vi "状态标记位读写.vi"(5 "更新状态？":bool, 7 "Slave ID":T2=enum."氨氮", 11 "状态":bool) -> (3 "流程运行状态标记位":T1)   [LabVIEW 2016, in "质控单元V4.lvlib"]
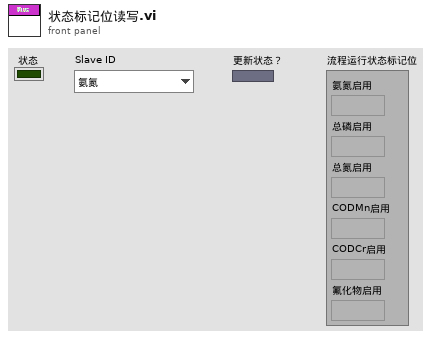
[diagram p1: front panel]
types:
  T1 = typedef "质控单元V4.lvlib/启动参数.ctl" = cluster{"氨氮启用":bool, "总磷启用":bool, "总氮启用":bool, "CODMn启用":bool, "CODCr启用":bool, "氟化物启用":bool}
  T2 = typedef "质控单元V4.lvlib/质控slave id.ctl" = enum16{"null", "氨氮", "总磷", "总氮", "CODMn", "CODCr", "氟化物", "挥发酚"}
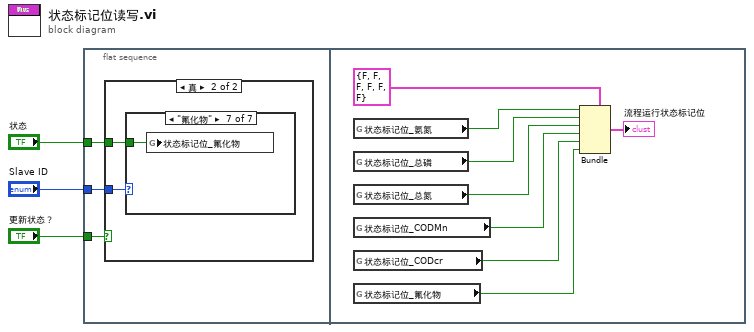
[diagram p0: block diagram]
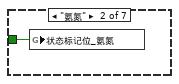
[diagram p4: hidden frame]
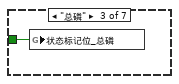
[diagram p5: hidden frame]
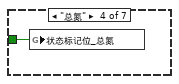
[diagram p6: hidden frame]
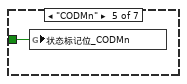
[diagram p7: hidden frame]
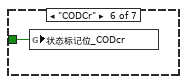
[diagram p8: hidden frame]
diagram:
  n1 = flat-sequence {
    tunnel: "Slave ID" -> [w6]
    tunnel: "状态" -> [w5]
    tunnel: "更新状态？" -> [w4]
    frame #0 {
      n2 = case shown="真" w4 {
        tunnel: w6 -> [_ w8]
        tunnel: w5 -> [_ w7]
        frame False {
        }
        frame True {
          n3 = case shown="\"氟化物\"" w8 {
            tunnel: w7 -> [_ w9 w10 w11 w12 w13 w14]
            frame "null", Default {
            }
            frame "氨氮" {
              n4 = global write "ZK非断电保存全局变量.vi" "状态标记位_氨氮"(w9) -> ()
            }
            frame "总磷" {
              n5 = global write "ZK非断电保存全局变量.vi" "状态标记位_总磷"(w10) -> ()
            }
            frame "总氮" {
              n6 = global write "ZK非断电保存全局变量.vi" "状态标记位_总氮"(w11) -> ()
            }
            frame "CODMn" {
              n7 = global write "ZK非断电保存全局变量.vi" "状态标记位_CODMn"(w12) -> ()
            }
            frame "CODCr" {
              n8 = global write "ZK非断电保存全局变量.vi" "状态标记位_CODcr"(w13) -> ()
            }
            frame "氟化物" {
              n9 = global write "ZK非断电保存全局变量.vi" "状态标记位_氟化物"(w14) -> ()
            }
          }
        }
      }
    }
    frame #1 {
      n10 = global read "ZK非断电保存全局变量.vi" "状态标记位_氨氮"() -> (w22:bool)
      n11 = global read "ZK非断电保存全局变量.vi" "状态标记位_总磷"() -> (w21:bool)
      n12 = global read "ZK非断电保存全局变量.vi" "状态标记位_总氮"() -> (w20:bool)
      n13 = global read "ZK非断电保存全局变量.vi" "状态标记位_CODMn"() -> (w19:bool)
      n14 = global read "ZK非断电保存全局变量.vi" "状态标记位_CODcr"() -> (w18:bool)
      n15 = global read "ZK非断电保存全局变量.vi" "状态标记位_氟化物"() -> (w15:bool)
      n16 = Bundle(cluster=T1 {"氨氮启用"=FALSE, "总磷启用"=FALSE, "总氮启用"=FALSE, "CODMn启用"=FALSE, "CODCr启用"=FALSE, "氟化物启用"=FALSE} ("流程运行状态标记位"), "氨氮启用"=w22, "总磷启用"=w21, "总氮启用"=w20, "CODMn启用"=w19, "CODCr启用"=w18, "氟化物启用"=w15) -> (→"流程运行状态标记位":T1)
    }
  }
